vi "List Tables.vi"(8 "error in (no error)":errorcluster, 10 "database":string, 11 "mysql in":refnum<class "mysql.lvclass">) -> (0 "error out":errorcluster, 2 "tables":string[](array[string]), 3 "mysql out":refnum<class "mysql.lvclass">)   [LabVIEW 2020, in "mysql.lvlib" / "mysql.lvclass"]
uses:
  mysql.lvclass
  33f63fa6-d95e-4f8b-90c2-49c7121e4c97.vi
  <vilib>/Utility/error.llb/Error Cluster From Error Code.vi
panel:
  out "tables info":string[][](array[string])
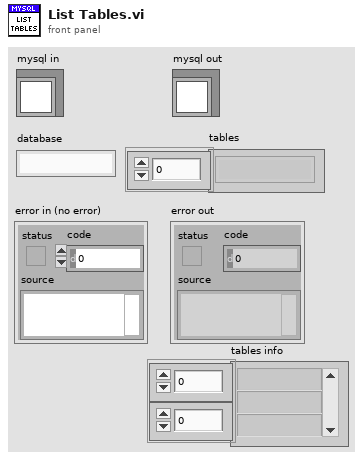
[diagram p1: front panel]
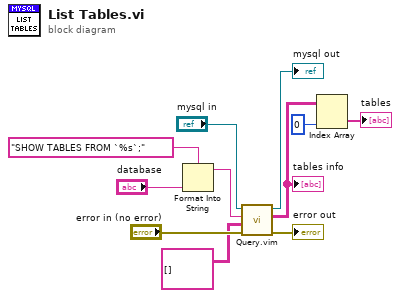
[diagram p0: block diagram]
diagram:
  n1 = Format Into String(format string="SHOW TABLES FROM `%s`;" ("Query string"), "database") -> (resulting string=w10:string)  [unwired: 2 in, 1 out]
  n2 = call "Query.vim"("error in (no error)"="error in (no error)", "Type and Default"=string[][] [] ("tables info 2"), "Query string"=w10, "IDatabase in"="mysql in") -> ("error out"=→"error out":errorcluster, "Result"=w9:string[][], "IDatabase out"=→"mysql out":refnum<class "mysql.lvclass">)  [unwired: 5 in]
  "tables info" <- w9
  n3 = Index Array(array=w9, index (col)=0 ("disabled index (col)")) -> (element=→"tables":string[])  [unwired: 1 in]
